vi "OAT IIR Preprocess Filter (1 Channel).vi"(0 "scaled signal [EU]":waveform(dbl)={"t0"=timestamp(0 s since 1904-01-01), "dt"=0.0, "Y"=[]}, 1 "filter type":T3(ring), 2 "reset? (F)":bool, 3 "design method":u16(ring) items=["Butterworth", "Chebyshev", "Inverse Chebyshev", "Elliptic"], 5 "order":i32=2 min=1, 7 "freq specs [Hz]":T2={"low cutoff freq"=100.0, "high cutoff freq"=200.0} {"high cutoff freq" format="%#.2f"; "low cutoff freq" format="%#.4f"}, 9 "ripple specs [dB]":T1={"passband ripple"=0.1, "stopband attenuation"=60.0} {"stopband attenuation" format="%#.2f"; "passband ripple" format="%#.2f"}, 11 "error in (no error)":errorcluster) -> (4 "filtered scaled signal [EU]":waveform(dbl), 15 "error out":errorcluster)   [LabVIEW 2017, in "SoundVib_RefDataProcess.lvlib"]
doc: "Designs an IIR filter and filters the <B>scaled signal [EU]</B>. Each instance of this VI maintains its own state; use the N Waveforms instance of this VI to process an array of channels. Wire data to the <B>scaled signal [EU]</B> input to determine the polymorphic instance to use or manually select the instance."
uses:
  <vilib>/addons/Sound and Vibration/Order Analysis/Referece Data Processing/SoundVib_RefDataProcess.lvlib
  <vilib>/addons/_NISVFA/_Shared subVIs/Common/svc_Check for Waveform Parameter Continuity (no state).vi
  <vilib>/addons/_NISVFA/_Shared subVIs/Common/svc_Get SV Channel Info.vi
  <vilib>/Analysis/baseanly.llb/IIR Cascade Filter (DBL).vi
  <vilib>/addons/_NISVFA/_Shared subVIs/Common/svc_Engineering Units to Unit Label.vi
  <vilib>/addons/_NISVFA/_Shared subVIs/Common/svc_Unit Label to Engineering Units.vi
  <vilib>/Analysis/NI_AALBase.lvlib
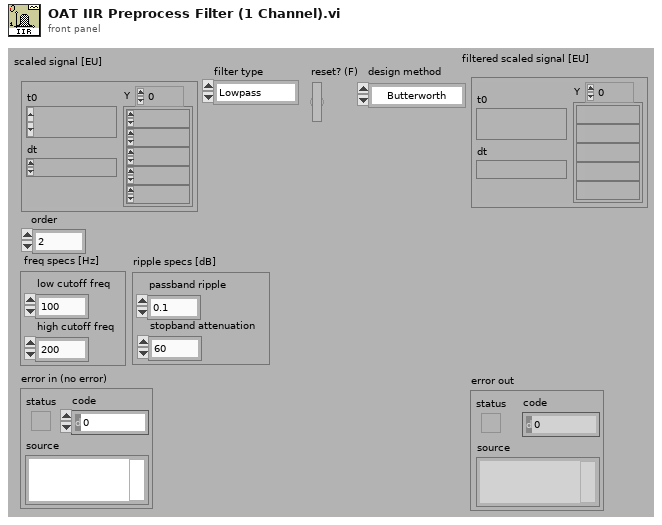
[diagram p1: front panel]
types:
  T1 = cluster{"passband ripple":dbl, "stopband attenuation":dbl}
  T2 = cluster{"low cutoff freq":dbl, "high cutoff freq":dbl}
  T3 = enum32{"Lowpass", "Highpass", "Bandpass", "Bandstop"}
  T4 = cluster{"dt":bool, "t0 continuity":bool, "array length":bool, "channel info":bool, "name":bool}
  T5 = cluster{"filter structure":enum32{"IIR 2nd Order", "IIR 4th Order"}, "Reverse Coefficients":dbl[], "Forward Coefficients":dbl[]}
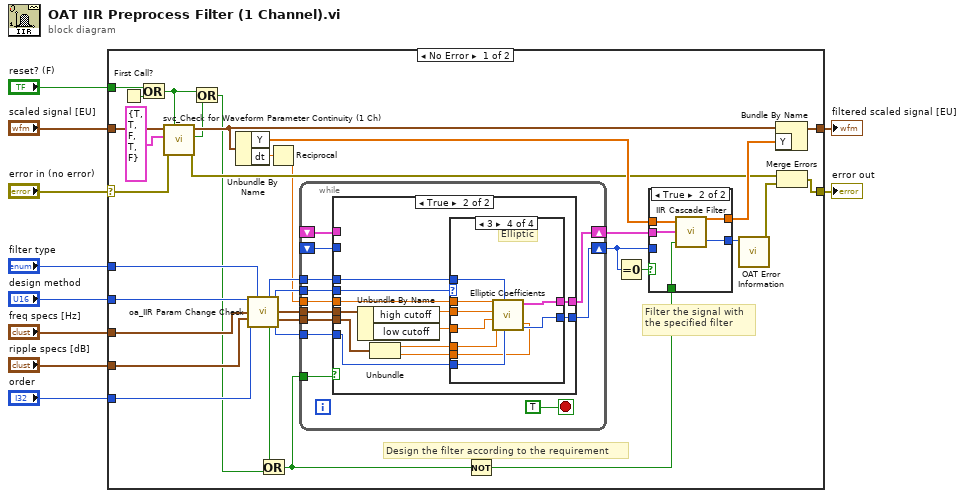
[diagram p0: block diagram]
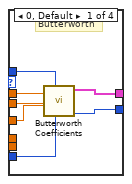
[diagram p3: hidden frame]
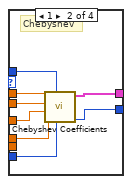
[diagram p4: hidden frame]
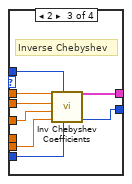
[diagram p5: hidden frame]
diagram:
  n1 = case shown="No Error" "error in (no error)" {
    selector: "error in (no error)" -> [w12 w110]
    tunnel: [w23 w110] -> w10
    tunnel: "scaled signal [EU]" -> [w22 w111]
    tunnel: [w41 w111] -> w4
    tunnel: "design method" -> [w38 _]
    tunnel: "filter type" -> [w26 _]
    tunnel: "freq specs [Hz]" -> [w30 _]
    tunnel: "ripple specs [dB]" -> [w29 _]
    tunnel: "order" -> [w28 _]
    tunnel: "reset? (F)" -> [w13 _]
    frame No Error {
      # "Design the filter according to the requirement"
      # "Filter the signal with \nthe specified filter"
      n2 = First Call?() -> (First Call?: T/F=w20:bool)
      n3 = Or(x=w13, y=w20) -> (x .or. y?=w16:bool)
      n4 = call <vilib>:"svc_Check for Waveform Parameter Continuity (1 Ch).vi"("restart averaging (F)"=w16, "error in (no error)"=w12, "checks for channel parameter change"=T4 {"dt"=TRUE, "t0 continuity"=TRUE, "array length"=FALSE, "channel info"=TRUE, "name"=FALSE}, "scaled signal [EU]"=w22) -> ("error out"=w18:errorcluster, "waveform parameter changed"=w17:bool, "dup scaled signal [EU]"=w21:waveform(dbl))  [unwired: 2 in, 3 out]
      n5 = Or(x=w16, y=w17) -> (x .or. y?=w15:bool)
      n6 = Unbundle By Name(w21) -> ("Y"=w40:dbl[], "dt"=w14:dbl)
      n7 = call <vilib>:"oa_IIR Param Change Check.vi"("design method in"=w38, "filter type in"=w26, "freq specs in"=w30, "ripple specs in [dB]"=w29, "order in"=w28) -> ("filter type out"=w37:T3, "design method out"=w36:u16, "freq specs out"=w32:cluster{"low cutoff":dbl, "high cutoff":dbl}, "ripple specs out [dB]"=w31:cluster{"pass band":dbl, "stop band":dbl}, "chang?"=w27:bool, "order out"=w33:i32)  [unwired: 4 in, 1 out]
      n8 = Or(x=w27, y=w15) -> (x .or. y?=w35:bool)
      n9 = Reciprocal(x=w14) -> (1/x=w11:dbl)
      n10 = while {
        tunnel: w35 -> [w54]
        shift-right: [w55] -> w39
        shift-left: _ -> [w52]
        shift-right: [w56] -> w43
        shift-left: _ -> [w51]
        tunnel: w36 -> [w50]
        tunnel: w37 -> [w49]
        tunnel: w32 -> [w48]
        tunnel: w31 -> [w47]
        tunnel: w33 -> [w46]
        tunnel: w11 -> [w45]
        stop <- TRUE stop-if-true
        n11 = case shown="True" w54 {
          tunnel: [w57 w70] -> w56
          tunnel: [w58 w69] -> w55
          tunnel: w52 -> [w58 _]
          tunnel: w51 -> [w57 _]
          tunnel: w50 -> [_ w68]
          tunnel: w49 -> [_ w67]
          tunnel: w48 -> [_ w64]
          tunnel: w47 -> [_ w63]
          tunnel: w46 -> [_ w66]
          tunnel: w45 -> [_ w65]
          frame False {
          }
          frame True {
            n12 = Unbundle By Name(w64) -> ("high cutoff"=w62:dbl, "low cutoff"=w61:dbl)
            n13 = Unbundle(w63) -> ("pass band"=w60:dbl, "stop band"=w59:dbl)
            n14 = case shown="3" w68 {
              tunnel: [w77 w85 w93 w102] -> w69
              tunnel: [w76 w84 w92 w101] -> w70
              tunnel: w67 -> [w75 w83 w91 w100]
              tunnel: w66 -> [w71 w78 w86 w95]
              tunnel: w65 -> [w74 w82 w90 w99]
              tunnel: w62 -> [w73 w81 w89 w98]
              tunnel: w61 -> [w72 w80 w88 w97]
              tunnel: w60 -> [_ w79 _ w96]
              tunnel: w59 -> [_ _ w87 w94]
              frame 0, Default {
                # "Butterworth"
                n15 = call <vilib>:"Butterworth Coefficients.vi"("order"=w71, "filter type"=w75, "low cutoff freq: fl"=w72, "high cutoff freq: fh"=w73, "sampling freq: fs"=w74) -> ("error"=w76:i32, "IIR Filter Cluster"=w77:T5)  [unwired: 5 in]
              }
              frame 1 {
                # "Chebyshev"
                n16 = call <vilib>:"Chebyshev Coefficients.vi"("order"=w78, "filter type"=w83, "ripple(dB)"=w79, "low cutoff freq: fl"=w80, "high cutoff freq: fh"=w81, "sampling freq: fs"=w82) -> ("error"=w84:i32, "IIR Filter Cluster"=w85:T5)  [unwired: 4 in]
              }
              frame 2 {
                # "Inverse Chebyshev"
                n17 = call <vilib>:"Inv Chebyshev Coefficients.vi"("order"=w86, "filter type"=w91, "attenuation (dB)"=w87, "low cutoff freq: fl"=w88, "high cutoff freq: fh"=w89, "sampling freq: fs"=w90) -> ("error"=w92:i32, "IIR Filter Cluster"=w93:T5)  [unwired: 4 in]
              }
              frame 3 {
                # "Elliptic"
                n18 = call <vilib>:"Elliptic Coefficients.vi"("stopband attenuation (dB)"=w94, "order"=w95, "filter type"=w100, "passband ripple (dB)"=w96, "low cutoff freq: fl"=w97, "high cutoff freq: fh"=w98, "sampling freq: fs"=w99) -> ("error"=w101:i32, "IIR Filter Cluster"=w102:T5)  [unwired: 3 in]
              }
            }
          }
        }
      }
      n19 = Not(x=w35) -> (.not. x?=w34:bool)
      n20 = Equal To 0?(x=w43) -> (x = 0?=w44:bool)
      n21 = case shown="True" w44 {
        tunnel: w43 -> [w104 _]
        tunnel: [w103 w107] -> w42
        tunnel: w39 -> [_ w109]
        tunnel: [w104 w108] -> w25
        tunnel: w40 -> [w103 w106]
        tunnel: w34 -> [_ w105]
        frame False {
        }
        frame True {
          n22 = call-poly <vilib>:"IIR Cascade Filter.vi"("init/cont (init:F)"=w105, "IIR Filter Cluster"=w109, "X"=w106) -> ("error"=w108:i32, "Filtered X"=w107:dbl[])
        }
      }
      n23 = call <vilib>:"OAT Error Information.vi"("error code"=w25) -> ("error out"=w24:errorcluster)  [unwired: 6 in]
      n24 = Bundle By Name(cluster=w21, "Y"=w42) -> (w41:waveform(dbl))
      n25 = Merge Errors(w18, w24) -> (w23:errorcluster)
    }
    frame Error {
    }
  }
  "error out" <- w10
  "filtered scaled signal [EU]" <- w4
